vi "VI Server Setup.vi"(9 "This VI":refnum<vi>, 10 "This Application":refnum<vi>, 11 "TEMPLATE Event in":refnum<class "TEMPLATE Event.lvclass">) -> (3 "TEMPLATE Event out":refnum<class "TEMPLATE Event.lvclass">)   [LabVIEW 2021, in "_Template.lvlib" / "Templates.lvlib" / "TEMPLATE Event.lvlib" / "TEMPLATE Event.lvclass"]
uses:
  TEMPLATE Event.lvclass
  TEMPLATE Event.lvclass/TEMPLATE Event.ctl
  <vilib>/Nathan Davis/jettl/jettl/Event/Event.lvclass
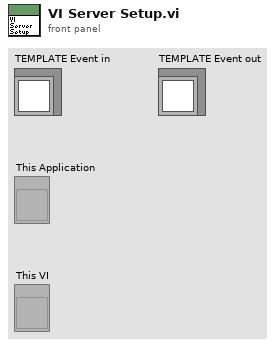
[diagram p1: front panel]
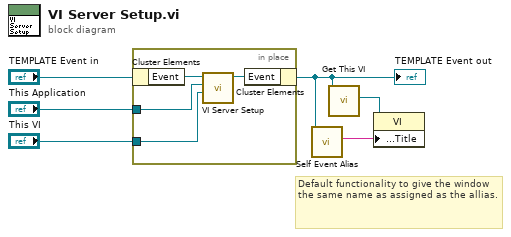
[diagram p0: block diagram]
diagram:
  # "Default functionality to give the window the same name as assigned as the allias."
  n1 = in-place {
    in-place-border: "This Application" -> [w8]
    in-place-border: "This VI" -> [w7]
    n2 = in-place-cluster #1("TEMPLATE Event in") -> ("Event"=w10:refnum<class "Event.lvclass">)
    n3 = call-dynamic "VI Server Setup.vi"("This VI"=w7, "This Application"=w8, "jettl in"=w10) -> ("jettl out"=w9:refnum<class "Event.lvclass">)  [unwired: 8 in]
    n4 = in-place-cluster #1("Event"=w9) -> (w3:refnum<class "TEMPLATE Event.lvclass">)
  }
  "TEMPLATE Event out" <- w3
  n5 = call-dynamic "Self Event Alias.vi"("TEMPLATE Event in"=w3) -> ("Self Event Alias"=w1:string)  [unwired: 10 in]
  n6 = call-dynamic "Get This VI.vi"("TEMPLATE Event in"=w3) -> ("This VI"=w2:refnum<vi>)  [unwired: 10 in]
  n7 = property class="VI"(reference=w2, "Front Panel.Title"=w1) -> ()  [unwired: 1 in, 2 out]
